vi "Set DDG External Output Time.vi"(8 "error in (no error)":errorcluster, 9 "uiWidth":cluster{}, 10 "uiDelay":cluster{}, 11 "uiIndex":u32) -> (0 "error out":errorcluster, 3 "function return":u32)   [LabVIEW 2014, in "atmcd32d.lvlib"]
doc: "unsigned int WINAPI SetDDGExternalOutputTime(at_u32 uiIndex, at_u64 uiDelay, at_u64 uiWidth);"
uses:
  atmcd32d.lvlib
  atmcd32d.dll
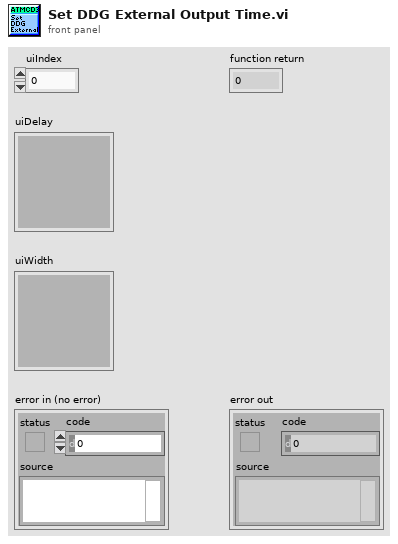
[diagram p1: front panel]
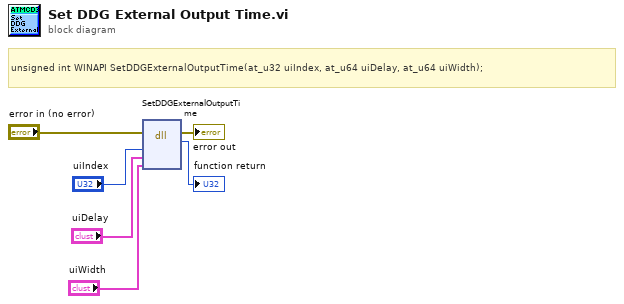
[diagram p0: block diagram]
diagram:
  # "unsigned int WINAPI SetDDGExternalOutputTime(at_u32 uiIndex, at_u64 uiDelay, at_u64 uiWidth);"
  n1 = dll-call lib="C:/Users/Bakir/Documents/Lambda2-Testing/lib/Andorlib/atmcd32d.*" fn="SetDDGExternalOutputTime"(error in="error in (no error)", "uiIndex"="uiIndex", "uiDelay"="uiDelay", "uiWidth"="uiWidth") -> (error out=→"error out":errorcluster, →"function return":u32)  [unwired: 5 in, 1 out]
